vi "DSF.Engine.Framework.Initialize Inline Buffer.vi"(8 "error in (no error)":errorcluster, 9 "channel count":u64, 10 "first channel offset":u64, 11 "Framework in":refnum<class "DSF.Engine.Framework.lvclass">) -> (0 "error out":errorcluster, 2 "Buffer":refnum<class "DSF.Engine.Pointer.DBL.lvclass">, 3 "Framework out":refnum<class "DSF.Engine.Framework.lvclass">)   [LabVIEW 2017, in "DSF.Engine.lvlib" / "DSF.Engine.Framework.lvclass"]
uses:
  DSF.Engine.Framework.lvclass
  Pointer/DSF.Engine.Pointer.DBL.lvclass
  DSF.Engine.Framework.lvclass/DSF.Engine.Framework.ctl
  Built/PharLap x86/Dependencies/c/Memory Manager.lvlibp/1abvi3w/vi.lib/National Instruments/Memory Manager/Classes/Pointer/Memory.Pointer.lvclass
  C:/Git/DSF/DSF Core/Built/Windows/Dependencies/Memory Manager.lvlibp/1abvi3w/vi.lib/National Instruments/Memory Manager/Classes/Pointer/Memory.Pointer.lvclass
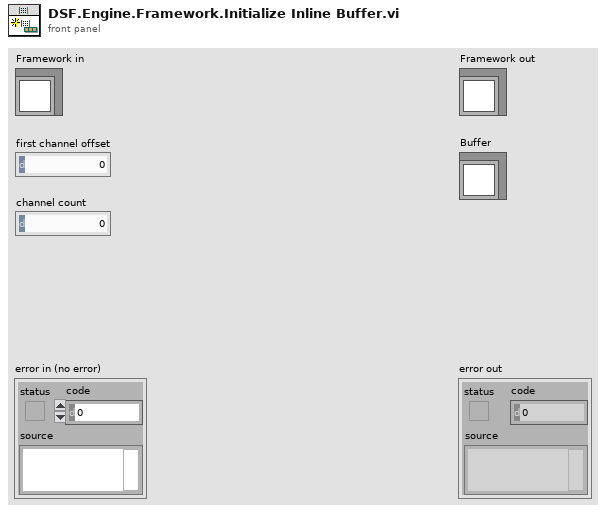
[diagram p1: front panel]
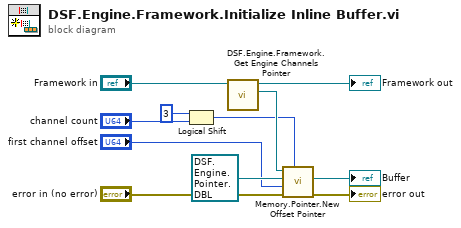
[diagram p0: block diagram]
diagram:
  n1 = Logical Shift(y=i16 3, x="channel count") -> (x << y=w2:u64)
  n2 = call "DSF.Engine.Framework.Get Engine Channels Pointer.vi"("Framework in"="Framework in") -> ("Engine Channels Pointer"=w6:refnum<class "DSF.Engine.Pointer.DBL.lvclass">, "Framework out"=→"Framework out":refnum<class "DSF.Engine.Framework.lvclass">)  [unwired: 9 in]
  n3 = call "Memory.Pointer.New Offset Pointer.vi"("length (-1: rest)"=w2, "error in (no error)"="error in (no error)", "offset (0)"="first channel offset", "offset Pointer type"=refnum<class "DSF.Engine.Pointer.DBL.lvclass"> refnum ("Buffer"), "base Pointer in"=w6) -> ("error out"=→"error out":errorcluster, "offset Pointer"=→"Buffer":refnum<class "DSF.Engine.Pointer.DBL.lvclass">)  [unwired: 3 in, 2 out]
